vi "87-176 (SubVI).vi"(3 "Input":string, 4 "Channel":dbl=1.0 min=1.0 step=1.0, 5 "Input":T1) -> (2 "Output":T1)   [LabVIEW 2024]
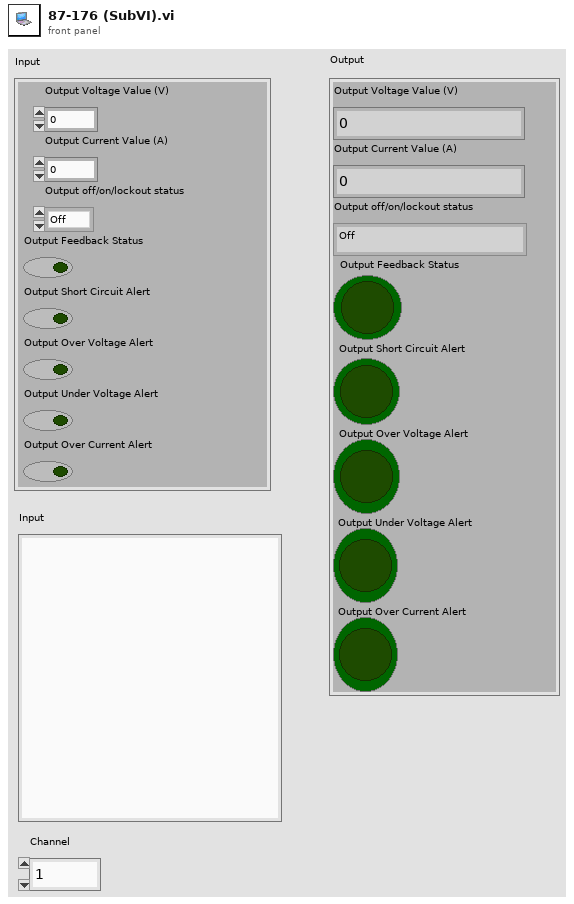
[diagram p1: front panel]
types:
  T1 = cluster{"Output Voltage Value (V)":dbl, "Output Current Value (A)":dbl, "Output off/on/lockout status":enum16{"Off", "On", "Lockout"}, "Output Feedback Status":bool, "Output Short Circuit Alert":bool, "Output Over Voltage Alert":bool, "Output Under Voltage Alert":bool, "Output Over Current Alert":bool}
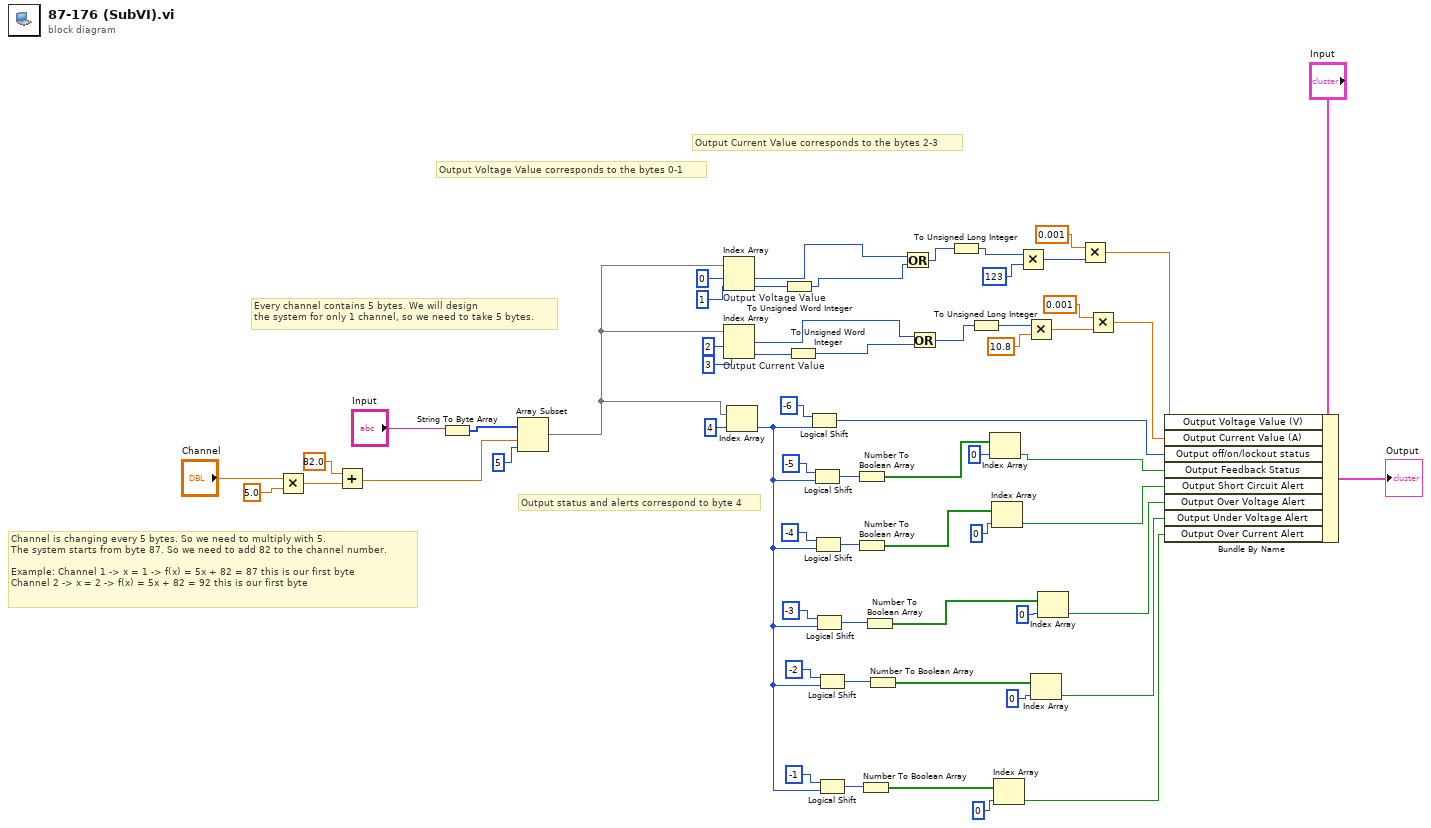
[diagram p0: block diagram]
diagram:
  # "Output status and alerts correspond to byte 4"
  # "Output Current Value corresponds to the bytes 2-3"
  # "Output Voltage Value corresponds to the bytes 0-1"
  # "Every channel contains 5 bytes. We will design \nthe system for only 1 channel, so we need to take 5 bytes."
  # "Channel is changing every 5 bytes. So we need to multiply with 5.\nThe system starts from byte 87. So we need to add 82 to the channel number.\n\nExample: Channel 1 -> x = 1 -> f(x) = 5x + 82 = 87 this is our first byte\nChannel 2 -> x = 2 -> f(x) = 5x + 82 = 92 this is our first byte"
  n1 = Multiply(x="Channel", y=5.0) -> (x*y=w3:dbl)
  n2 = Add(x=82.0, y=w3) -> (x+y=w31:dbl)
  n3 = String To Byte Array(string="Input") -> (unsigned byte array=w29:u8[])
  n4 = Array Subset(array=w29, index=w31, length=5) -> (w32:u8[])
  n5 = Index Array "Output Voltage Value"(array=w32, index #1=0 ("index"), index #2=1 ("index")) -> (element #1=w12:u8, element #2=w10:u8)
  n6 = Index Array "Output Current Value"(array=w32, index #1=2 ("index"), index #2=3 ("index")) -> (element #1=w13:u8, element #2=w11:u8)
  n7 = Index Array(array=w32, index=4) -> (element=w42:u8)
  n8 = To Unsigned Word Integer(number=w10) -> (unsigned 16bit integer=w37:u16)
  n9 = To Unsigned Word Integer(number=w11) -> (unsigned 16bit integer=w38:u16)
  n10 = Logical Shift(y=i16 -6, x=w42) -> (x << y=w55:u8)
  n11 = Logical Shift(y=i16 -5, x=w42) -> (x << y=w22:u8)
  n12 = Logical Shift(y=i16 -4, x=w42) -> (x << y=w24:u8)
  n13 = Logical Shift(y=i16 -3, x=w42) -> (x << y=w39:u8)
  n14 = Logical Shift(y=i16 -2, x=w42) -> (x << y=w41:u8)
  n15 = Logical Shift(y=i16 -1, x=w42) -> (x << y=w27:u8)
  n16 = Number To Boolean Array(number=w22) -> (Boolean array=w43:bool[])
  n17 = Number To Boolean Array(number=w24) -> (Boolean array=w49:bool[])
  n18 = Number To Boolean Array(number=w27) -> (Boolean array=w52:bool[])
  n19 = Number To Boolean Array(number=w39) -> (Boolean array=w50:bool[])
  n20 = Number To Boolean Array(number=w41) -> (Boolean array=w51:bool[])
  n21 = Or(x=w12, y=w37) -> (x .or. y?=w33:u16)
  n22 = Or(x=w13, y=w38) -> (x .or. y?=w35:u16)
  n23 = To Unsigned Long Integer(number=w33) -> (unsigned 32bit integer=w34:u32)
  n24 = To Unsigned Long Integer(number=w35) -> (unsigned 32bit integer=w36:u32)
  n25 = Index Array(array=w43, index=0) -> (element=w56:bool)
  n26 = Index Array(array=w49, index=0) -> (element=w57:bool)
  n27 = Index Array(array=w52, index=0) -> (element=w60:bool)
  n28 = Multiply(x=w34, y=u32 123) -> (x*y=w15:u32)
  n29 = Multiply(x=w36, y=10.8) -> (x*y=w18:dbl)
  n30 = Index Array(array=w51, index=0) -> (element=w59:bool)
  n31 = Index Array(array=w50, index=0) -> (element=w58:bool)
  n32 = Multiply(x=0.001, y=w15) -> (x*y=w53:dbl)
  n33 = Multiply(x=0.001, y=w18) -> (x*y=w54:dbl)
  n34 = Bundle By Name(cluster="Input", "Output Voltage Value (V)"=w53, "Output Current Value (A)"=w54, "Output off/on/lockout status"=w55, "Output Feedback Status"=w56, "Output Short Circuit Alert"=w57, "Output Over Voltage Alert"=w58, "Output Under Voltage Alert"=w59, "Output Over Current Alert"=w60) -> (→"Output":T1)
